vi "create waveform sub.vi"(10 "amplitude":dbl, 11 "index":i32) -> (3 "Array":dbl[](array[numeric]))   [LabVIEW 2014]
uses:
  <vilib>/measure/NI_MAPro.lvlib
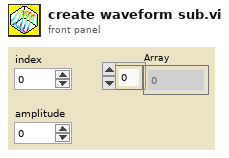
[diagram p1: front panel]
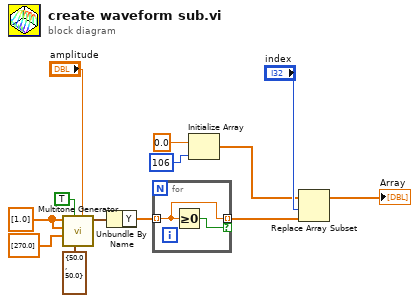
[diagram p0: block diagram]
diagram:
  w7 = dbl[] [1.0] ("tone frequencies")
  n1 = call <vilib>:"Multitone Generator.vi"("amplitude"="amplitude", "sampling info"=cluster{"Fs":dbl, "#s":dbl} {"Fs"=50.0, "#s"=50.0}, "reset signal"=TRUE, "tone phases"=dbl[] [270.0], "tone amplitudes"=w7, "tone frequencies"=w7) -> ("signal out"=w5:waveform(dbl))  [unwired: 2 in, 3 out]
  n2 = Unbundle By Name(w5) -> ("Y"=w6:dbl[])
  n3 = for {
    tunnel: w6 -> [w14] mode=indexing
    tunnel: [w14] -> w13 mode=indexing if=w15
    n4 = Greater Or Equal To 0?(x=w14) -> (x >= 0?=w15:bool)
  }
  n5 = Initialize Array(0.0 ("amplitude"), 106 ("dimension size")) -> (w10:dbl[])
  n6 = Replace Array Subset(array=w10, new element=w13, index="index") -> (→"Array":dbl[])
